vi "Get Section ID.vi"(6 "User Email":string="myemail", 7 "Notebook Name":string="My notebook on One Drive", 8 "Error In (No Error)":errorcluster, 9 "Year (Section Group)":string, 10 "Month (Section)":string, 11 "client handle":T1) -> (0 "error out":errorcluster, 2 "Section ID":string, 3 "client handle out":T1)   [LabVIEW 2019, in "OneNote Library.lvlib"]
uses:
  OneNote Library.lvlib
  <vilib>/httpClient/ClientHandle.ctl
  <vilib>/JDP Science/JSONtext/String Subset.vi
  <vilib>/JDP Science/JSONtext/support/Strip Quotes and Unescape.vi
  <vilib>/JDP Science/JSONtext/support/Unescape JSON string.vi
  <vilib>/JDP Science/JSONtext/Parsing/Parse Full Path or Item Name.vi
  <vilib>/JDP Science/JSONtext/Offset/Find Item Locations by Path.vi
  Useful OAuth VIs/globals.vi
  <vilib>/httpClient/POSTBuffer.vi
  <vilib>/JDP Science/JSONtext/Next JSON Value.vi
  <vilib>/JDP Science/JSONtext/support/Error Cluster From Code.vi
  <vilib>/httpClient/LabVIEWHTTPClient.lvlib
  <vilib>/JDP Science/JSONtext/JSONtext.lvlib
  Useful HTTP VIs/Useful HTTP VIs.lvlib
  Useful OAuth VIs/Useful OAuth VIs.lvlib
panel:
  out "body 2":string
  out "key not found?":bool
  out "map":map{string, string}(c390)
  out "Request URI":string caption="Result"
  out "body":string
  out "headers":string
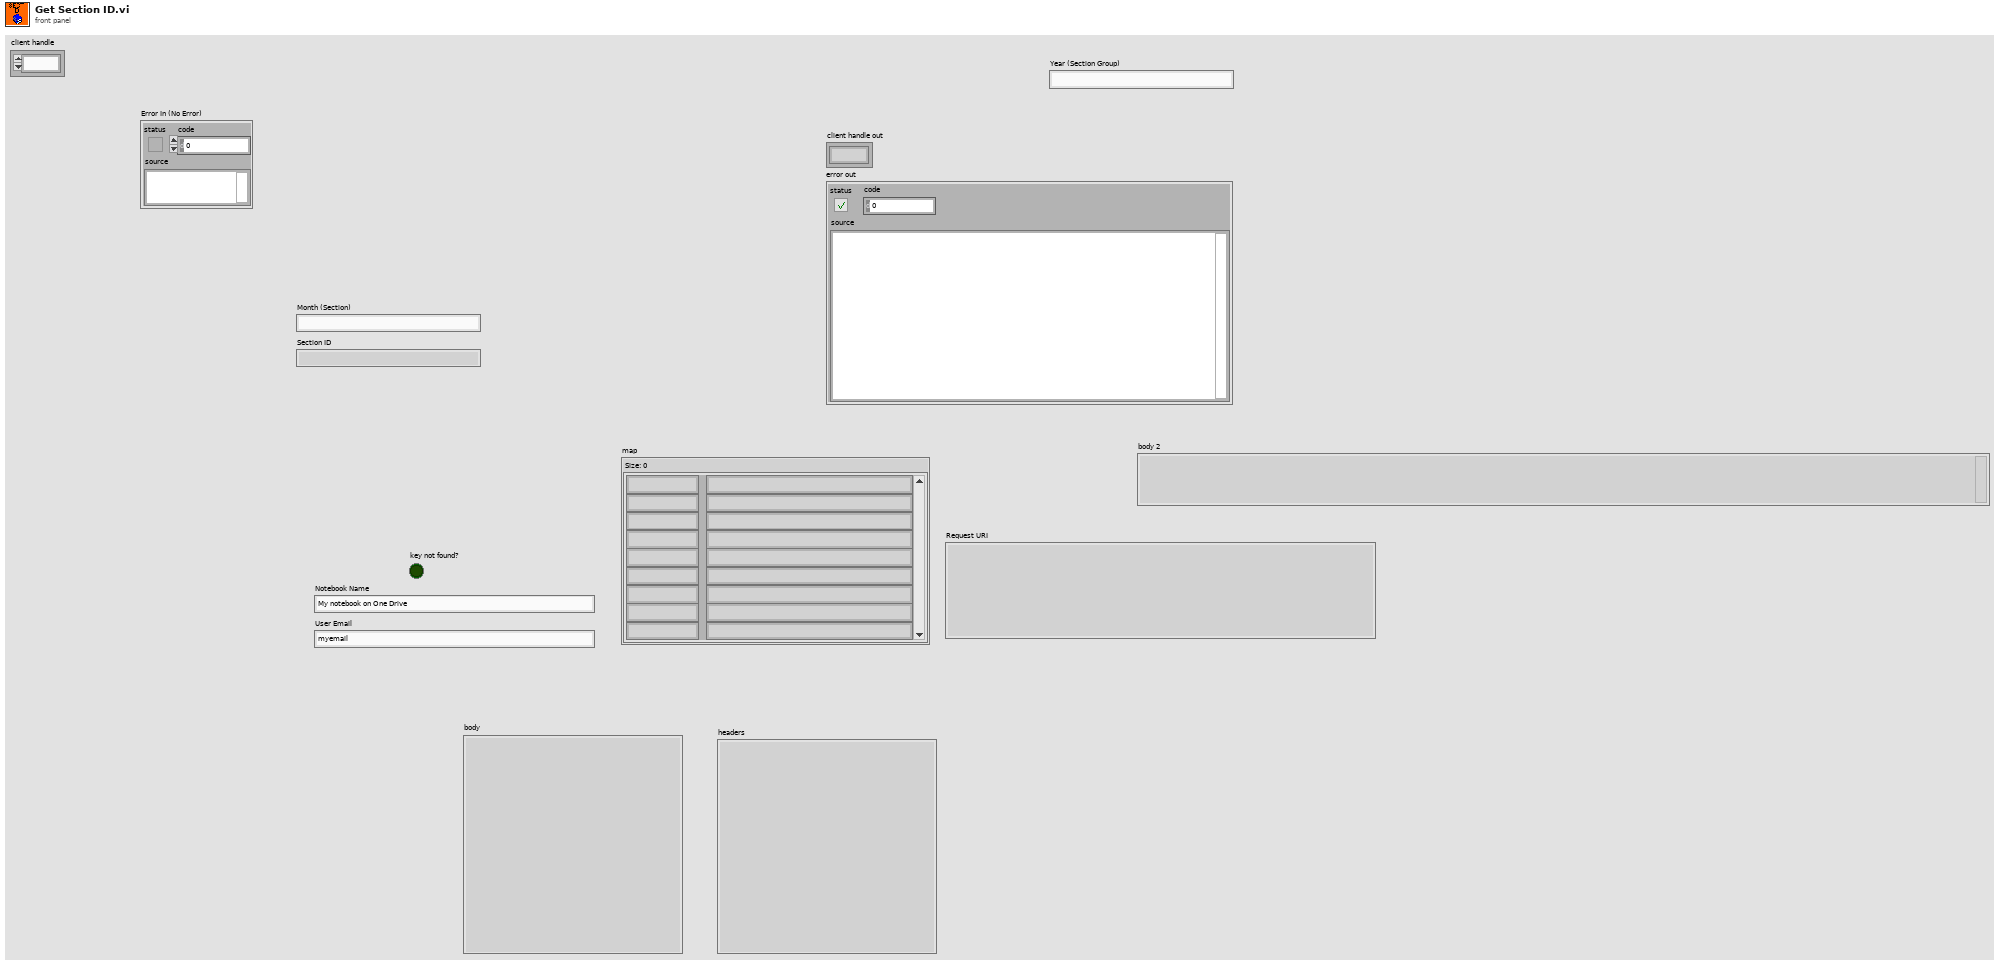
[diagram p1: front panel]
types:
  T1 = typedef "LabVIEWHTTPClient.lvlib/ClientHandle.ctl" = refnum<k1>
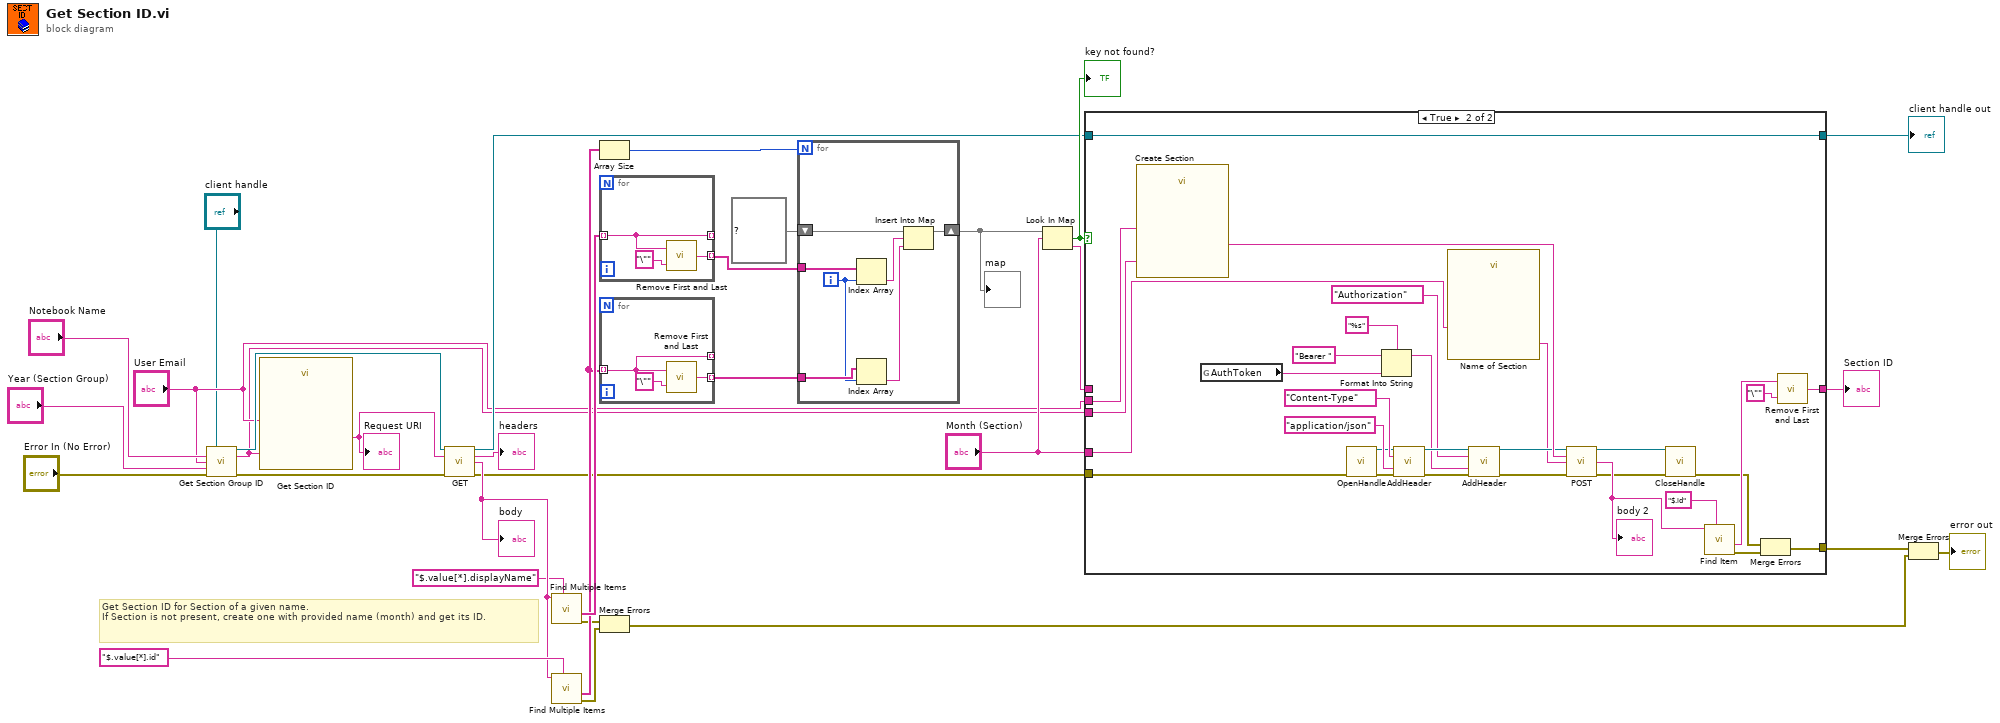
[diagram p0: block diagram]
diagram:
  # "Get Section ID for Section of a given name. \nIf Section is not present, create one with provided name (month) and get its ID."
  n1 = call "Get Section Group ID.vi"("client handle"="client handle", "Notebook Name"="Notebook Name", "User Email"="User Email", "Year (Section Group)"="Year (Section Group)", "Error In (No Error)"="Error In (No Error)") -> ("client handle out"=w6:T1, "Section Group ID"=w2:string, "error out"=w7:errorcluster)  [unwired: 8 in]
  n2 = call "Get Section ID"("user"="User Email", "Section Group ID"=w2) -> ("Result"=w32:string)  [unwired: 12 in, 1 out]
  "Request URI" <- w32
  n3 = call <vilib>:"GET.vi"("client handle"=w6, "url"=w32, "error in (no error)"=w7) -> ("client handle out"=w16:T1, "headers"=→"headers":string, "body"=w29:string, "error out"=w14:errorcluster)  [unwired: 9 in]
  "body" <- w29
  n4 = call <vilib>:"Find Multiple Items.vi"("$Path or Item Name"="$.value[*].displayName", "JSON"=w29) -> ("error out"=w13:errorcluster, "<JSON>"=w27:string[])  [unwired: 6 in, 2 out]
  n5 = call <vilib>:"Find Multiple Items.vi"("$Path or Item Name"="$.value[*].id", "JSON"=w29) -> ("error out"=w12:errorcluster, "<JSON>"=w23:string[])  [unwired: 6 in, 2 out]
  n6 = Array Size(array=w23) -> (size(s)=w22:i32)
  n7 = for {
    tunnel: w27 -> [w33] mode=indexing
    tunnel: [w33] -> _ mode=indexing
    tunnel: [w34] -> w26 mode=indexing
    n8 = call "Remove First and Last.vi"("Char to Remove"="\"", "String"=w33) -> ("Result"=w34:string)
  }
  n9 = for {
    tunnel: w23 -> [w36] mode=indexing
    tunnel: [w36] -> _ mode=indexing
    tunnel: [w37] -> w25 mode=indexing
    n10 = call "Remove First and Last.vi"("Char to Remove"="\"", "String"=w36) -> ("Result"=w37:string)
  }
  n11 = Merge Errors(w13, w12) -> (w10:errorcluster)
  n12 = for {
    N: w22 -> [_]
    tunnel: w25 -> [w45]
    tunnel: w26 -> [w44]
    shift-right: [w41] -> w21
    shift-left: map{string, string} {} ("map") -> [w43]
    i -> [w42]
    n13 = Index Array(array=w44, index=w42) -> (element=w40:string)
    n14 = Index Array(array=w45, index=w42) -> (element=w39:string)
    n15 = Insert Into Map(map in=w43, key=w40, value=w39) -> (map out=w41:map{string, string})  [unwired: 2 out]
  }
  "map" <- w21
  n16 = Look In Map(map=w21, key="Month (Section)") -> (key not found?=w20:bool, value=w18:string)  [unwired: 1 in]
  "key not found?" <- w20
  n17 = case shown="True" w20 {
    tunnel: "User Email" -> [_ w78]
    tunnel: "Month (Section)" -> [_ w66]
    tunnel: w18 -> [w48 _]
    tunnel: [w48 w57] -> w17
    tunnel: [w46 w52] -> w11
    tunnel: w16 -> [w47 w55]
    tunnel: [w47 w55] -> w15
    tunnel: w14 -> [w46 w54]
    tunnel: w2 -> [_ w49]
    frame False {
    }
    frame True {
      n18 = call "Create Section"("User Email"=w78, "Section Group ID"=w49) -> ("Result"=w77:string)  [unwired: 12 in, 1 out]
      n19 = global read "globals.vi" "AuthToken"() -> (w68:string)
      n20 = call <vilib>:"OpenHandle.vi"("error in (no error)"=w54) -> ("client handle out"=w74:T1, "error out"=w60:errorcluster)  [unwired: 13 in]
      n21 = Format Into String(format string="%s", initial string="Bearer ", w68) -> (resulting string=w67:string)  [unwired: 1 in, 1 out]
      n22 = call <vilib>:"AddHeader.vi"("client handle"=w74, "header"="Content-Type", "value"="application/json", "error in (no error)"=w60) -> ("client handle out"=w73:T1, "error out"=w61:errorcluster)  [unwired: 10 in]
      n23 = call "Name of Section"("Month"=w66) -> ("Result"=w65:string)  [unwired: 13 in, 1 out]
      n24 = call <vilib>:"AddHeader.vi"("client handle"=w73, "header"="Authorization", "value"=w67, "error in (no error)"=w61) -> ("client handle out"=w71:T1, "error out"=w62:errorcluster)  [unwired: 10 in]
      n25 = call-poly <vilib>:"POST.vi"("client handle"=w71, "url"=w77, "buffer"=w65, "error in (no error)"=w62) -> ("client handle out"=w56:T1, "body"=w64:string, "error out"=w51:errorcluster)  [unwired: 8 in, 1 out]
      "body 2" <- w64
      n26 = call <vilib>:"CloseHandle.vi"("client handle"=w56, "error in (no error)"=w51) -> ("error out"=w50:errorcluster)  [unwired: 13 in]
      n27 = call <vilib>:"Find Item.vi"("$Path or Item Name"="$.id", "JSON"=w64) -> ("error out"=w53:errorcluster, "<JSON>"=w58:string)  [unwired: 6 in, 2 out]
      n28 = Merge Errors(w50, w53) -> (w52:errorcluster)
      n29 = call "Remove First and Last.vi"("Char to Remove"="\"", "String"=w58) -> ("Result"=w57:string)
    }
  }
  "Section ID" <- w17
  "client handle out" <- w15
  n30 = Merge Errors(w11, w10) -> (→"error out":errorcluster)
